vi "Create Font by Name Size and Style.vi"(8 "error in (no error)":errorcluster caption="错误输入（无错误）", 9 "style":i32(ring) items=["Regular"=0, "Bold"=1, "Italic"=2, "Underline"=4, "Strikeout"=8], 10 "emSize":sgl, 11 "familyName":string) -> (0 "error out":errorcluster caption="错误输出", 3 "新引用":refnum<k24>)   [LabVIEW 2011, in "Font.lvclass"]
uses:
  Font.lvclass
  System.Drawing
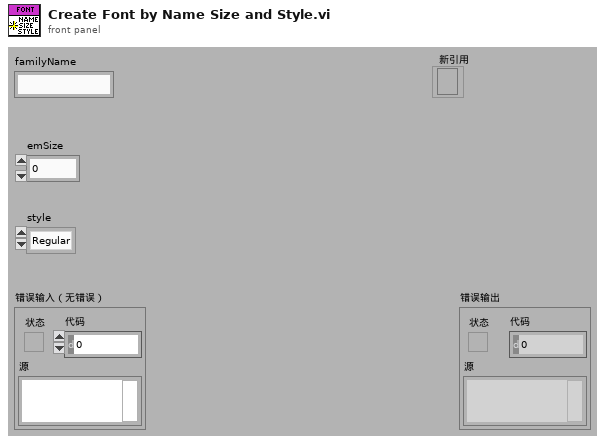
[diagram p1: front panel]
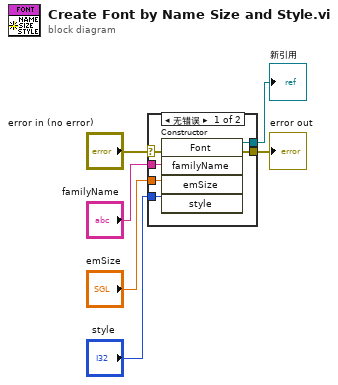
[diagram p0: block diagram]
diagram:
  n1 = case shown="无错误" "error in (no error)" {
    selector: "error in (no error)" -> [w12 w13]
    tunnel: [w11 w13] -> w5
    tunnel: "familyName" -> [w10 _]
    tunnel: "emSize" -> [w9 _]
    tunnel: "style" -> [w8 _]
    tunnel: [w7 _] -> w1
    frame No Error {
      n2 = constructor class="Font"(error in=w12, "familyName"=w10, "emSize"=w9, "style"=w8) -> (reference out=w7:refnum<k24>, error out=w11:errorcluster)  [unwired: 2 in, 4 out]
    }
    frame Error {
    }
  }
  "error out" <- w5
  "新引用" <- w1
